vi "output.vi"(8 "error in":errorcluster, 10 "data table in":T1, 11 "SQLite runtime in":refnum<class "SQLite runtime.lvclass">) -> (0 "error out":errorcluster, 2 "data table out":T1, 3 "SQLite runtime out":refnum<class "SQLite runtime.lvclass">)   [LabVIEW 2014, in "SQLite runtime.lvclass"]
doc: "Provides an interface for writing data to a module at runtime. While this interface performs no operations, a child should provide an override which may write to any open sessions, references, or interfaces."
uses:
  SQLite runtime.lvclass
  <vilib>/NI/Tag Bus/table/data table.ctl
  SQLite runtime.lvclass/SQLite runtime.ctl
  <vilib>/drjdpowell/SQLite Library/SQL Statement/SQL Statement.lvclass/SQL Statement.ctl
  <vilib>/NI/Tag Bus/table/data polymorphs/read one/read Double.vi
  <vilib>/NI/Tag Bus/table/data polymorphs/read one/read Single.vi
  <vilib>/drjdpowell/SQLite Library/SQL Statement/Bind Real.vi
  <vilib>/NI/Tag Bus/table/data polymorphs/read one/read I64.vi
  <vilib>/NI/Tag Bus/table/data polymorphs/read one/read I32.vi
  <vilib>/NI/Tag Bus/table/data polymorphs/read one/read I16.vi
  <vilib>/NI/Tag Bus/table/data polymorphs/read one/read I8.vi
  <vilib>/NI/Tag Bus/table/data polymorphs/read one/read U64.vi
  <vilib>/NI/Tag Bus/table/data polymorphs/read one/read U32.vi
  <vilib>/NI/Tag Bus/table/data polymorphs/read one/read U16.vi
  <vilib>/NI/Tag Bus/table/data polymorphs/read one/read U8.vi
  <vilib>/NI/Tag Bus/table/data polymorphs/read one/read Boolean.vi
  <vilib>/drjdpowell/SQLite Library/SQL Statement/Bind Integer.vi
  <vilib>/NI/Tag Bus/table/data polymorphs/read one/read String.vi
  <vilib>/drjdpowell/SQLite Library/SQL Statement/Bind Text.vi
  <vilib>/drjdpowell/SQLite Library/SQL Statement/First Step.vi
  <vilib>/drjdpowell/SQLite Library/SQL Statement/Reset (Property).vi
  <vilib>/drjdpowell/SQLite Library/SQL Statement/Step.vi
  <vilib>/drjdpowell/SQLite Library/SQL Statement/Reset.vi
  <vilib>/drjdpowell/SQLite Library/SQL Statement/Error Message.vi
  <vilib>/drjdpowell/SQLite Library/SQL Statement/SQL.vi
  <vilib>/NI/Tag Bus/table/data table.lvlib
  <vilib>/drjdpowell/SQLite Library/SQL Statement/SQL Statement.lvclass
panel:
  out "SQL 2":string
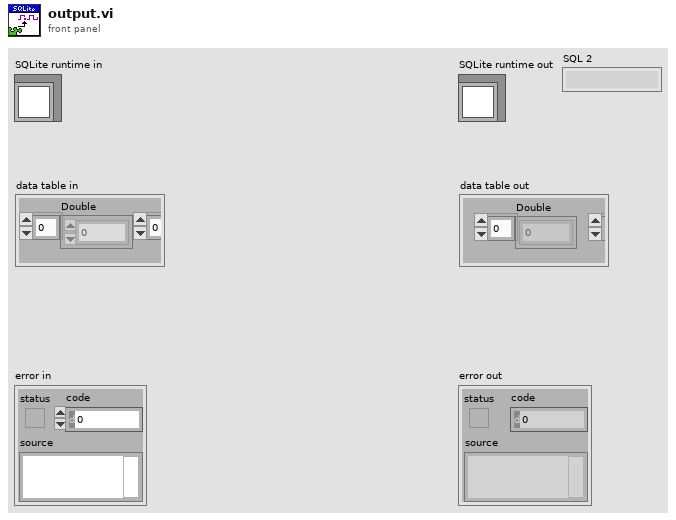
[diagram p1: front panel]
types:
  T1 = typedef "tag bus.lvlib/data table.lvlib/data table.ctl" = cluster{"Double":dbl[], "Single":sgl[], "I64":i64[], "I32":i32[], "I16":i16[], "I8":i8[], "U64":u64[], "U32":u32[], "U16":u16[], "U8":u8[], "Boolean":bool[], "String":string[], "Array of Double":cluster{"DBL Array":dbl[]}[], "Array of Single":cluster{"SGL Array":sgl[]}[], "Array of I64":cluster{"I64 Array":i64[]}[], "Array of I32":cluster{"I32 Array":i32[]}[], "Array of I16":cluster{"I16 Array":i16[]}[], "Array of I8":cluster{"I8 Array":i8[]}[], "Array of U64":cluster{"U64 Array":u64[]}[], "Array of U32":cluster{"U32 Array":u32[]}[], "Array of U16":cluster{"U16 Array":u16[]}[], "Array of U8":cluster{"U8 Array":u8[]}[], "Array of Boolean":cluster{"Boolean Array":bool[]}[], "Array of String":cluster{"String Array":string[]}[]}
  T2 = typedef "SQLite runtime.lvclass/data map.ctl" = cluster{"DCAF Type":T3, "Index":i32, "SQLite Type":T4, "db key":string}
  T3 = typedef "tag bus.lvlib/tag descriptor.lvclass/Data Type.ctl" = enum16{"Double", "Single", "I64", "I32", "I16", "I8", "U64", "U32", "U16", "U8", "Boolean", "String", "Array of Double", "Array of Single", "Array of I64", "Array of I32", "Array of I16", "Array of I8", "Array of U64", "Array of U32", "Array of U16", "Array of U8", "Array of Boolean", "Array of String"}
  T4 = typedef "SQLite runtime.lvclass/sqlite type.ctl" = enum16{"DBL", "I64", "String"}
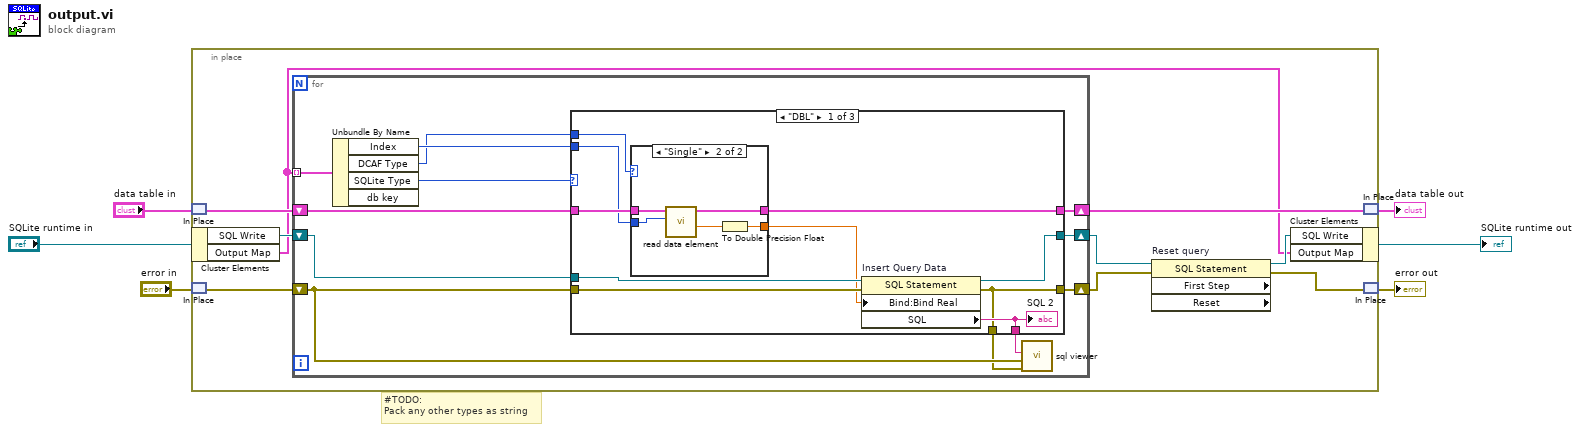
[diagram p0: block diagram]
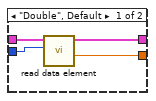
[diagram p2: hidden frame]
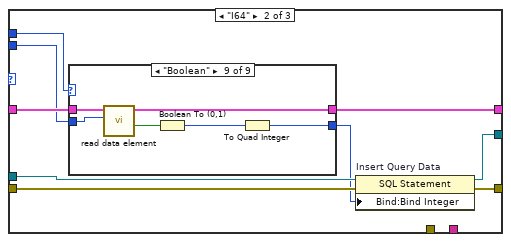
[diagram p3: hidden frame]
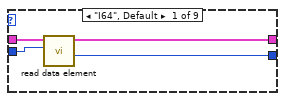
[diagram p4: hidden frame]
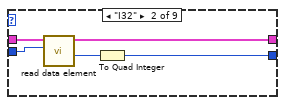
[diagram p5: hidden frame]
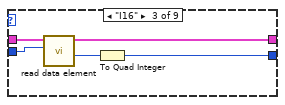
[diagram p6: hidden frame]
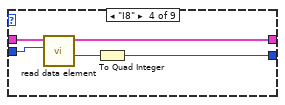
[diagram p7: hidden frame]
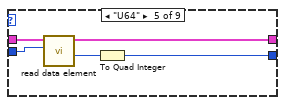
[diagram p8: hidden frame]
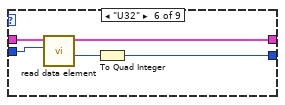
[diagram p9: hidden frame]
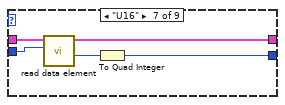
[diagram p10: hidden frame]
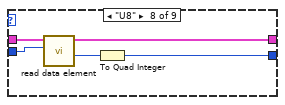
[diagram p11: hidden frame]
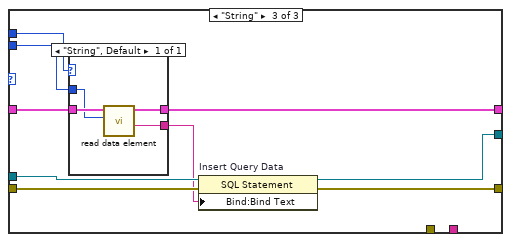
[diagram p12: hidden frame]
diagram:
  # "#TODO:\nPack any other types as string"
  n1 = in-place {
    n2 = in-place-match #1("data table in") -> (w11:T1)
    n3 = in-place-cluster #2("SQLite runtime in") -> ("SQL Write"=w15:refnum<class "SQL Statement.lvclass">, "Output Map"=w9:T2[])
    n4 = in-place-match #3("error in") -> (w14:errorcluster)
    n5 = for {
      shift-right: [w20] -> w7
      shift-left: w15 -> [w19]
      shift-right: [w21] -> w8
      shift-left: w14 -> [w18]
      shift-right: [w23] -> w10
      shift-left: w11 -> [w24]
      tunnel: w9 -> [w27] mode=indexing
      n6 = Unbundle By Name(w27) -> ("Index"=w25:i32, "DCAF Type"=w22:T3, "SQLite Type"=w26:T4)  [unwired: 1 out]
      n7 = case shown="\"DBL\"" w26 {
        tunnel: w19 -> [w37 w55 w109]
        tunnel: [w36 w48 w108] -> w20
        tunnel: w18 -> [w35 w54 w107]
        tunnel: [w28 w53 w106] -> w21
        tunnel: w25 -> [w31 w49 w103]
        tunnel: w24 -> [w34 w52 w105]
        tunnel: [w33 w51 w104] -> w23
        tunnel: w22 -> [w32 w50 w102]
        tunnel: [w29 _ _] -> w17
        tunnel: [w28 _ _] -> w16
        frame "DBL" {
          n8 = case shown="\"Single\"" w32 {
            tunnel: w34 -> [w41 w46]
            tunnel: [w40 w45] -> w33
            tunnel: w31 -> [w39 w44]
            tunnel: [w38 w42] -> w30
            frame "Double", Default {
              n9 = call-poly <vilib>:"read data element.vi"("index"=w39, "data table in"=w41) -> ("value"=w38:dbl, "data table out"=w40:T1)  [unwired: 8 in]
            }
            frame "Single" {
              n10 = call-poly <vilib>:"read data element.vi"("index"=w44, "data table in"=w46) -> ("value"=w43:sgl, "data table out"=w45:T1)  [unwired: 8 in]
              n11 = To Double Precision Float(number=w43) -> (double precision float=w42:dbl)
            }
          }
          n12 = property on="Insert Query Data" class="SQL Statement"(reference=w37, error in=w35, "Bind:Bind Real"=w30) -> (reference out=w36:refnum<class "SQL Statement.lvclass">, error out=w28:errorcluster, "SQL"=w29:string)
          "SQL 2" <- w29
        }
        frame "I64" {
          n13 = case shown="\"Boolean\"" w50 {
            tunnel: w52 -> [w59 w64 w69 w74 w79 w84 w89 w94 w100]
            tunnel: [w58 w63 w68 w73 w78 w83 w88 w93 w99] -> w51
            tunnel: w49 -> [w57 w62 w67 w72 w77 w82 w87 w92 w98]
            tunnel: [w56 w60 w65 w70 w75 w80 w85 w90 w95] -> w47
            frame "I64", Default {
              n14 = call-poly <vilib>:"read data element.vi"("index"=w57, "data table in"=w59) -> ("value"=w56:i64, "data table out"=w58:T1)  [unwired: 8 in]
            }
            frame "I32" {
              n15 = call-poly <vilib>:"read data element.vi"("index"=w62, "data table in"=w64) -> ("value"=w61:i32, "data table out"=w63:T1)  [unwired: 8 in]
              n16 = To Quad Integer(1:w61) -> (0:w60:i64)
            }
            frame "I16" {
              n17 = call-poly <vilib>:"read data element.vi"("index"=w67, "data table in"=w69) -> ("value"=w66:i16, "data table out"=w68:T1)  [unwired: 8 in]
              n18 = To Quad Integer(1:w66) -> (0:w65:i64)
            }
            frame "I8" {
              n19 = call-poly <vilib>:"read data element.vi"("index"=w72, "data table in"=w74) -> ("value"=w71:i8, "data table out"=w73:T1)  [unwired: 8 in]
              n20 = To Quad Integer(1:w71) -> (0:w70:i64)
            }
            frame "U64" {
              n21 = call-poly <vilib>:"read data element.vi"("index"=w77, "data table in"=w79) -> ("value"=w76:u64, "data table out"=w78:T1)  [unwired: 8 in]
              n22 = To Quad Integer(1:w76) -> (0:w75:i64)
            }
            frame "U32" {
              n23 = call-poly <vilib>:"read data element.vi"("index"=w82, "data table in"=w84) -> ("value"=w81:u32, "data table out"=w83:T1)  [unwired: 8 in]
              n24 = To Quad Integer(1:w81) -> (0:w80:i64)
            }
            frame "U16" {
              n25 = call-poly <vilib>:"read data element.vi"("index"=w87, "data table in"=w89) -> ("value"=w86:u16, "data table out"=w88:T1)  [unwired: 8 in]
              n26 = To Quad Integer(1:w86) -> (0:w85:i64)
            }
            frame "U8" {
              n27 = call-poly <vilib>:"read data element.vi"("index"=w92, "data table in"=w94) -> ("value"=w91:u8, "data table out"=w93:T1)  [unwired: 8 in]
              n28 = To Quad Integer(1:w91) -> (0:w90:i64)
            }
            frame "Boolean" {
              n29 = call-poly <vilib>:"read data element.vi"("index"=w98, "data table in"=w100) -> ("value"=w97:bool, "data table out"=w99:T1)  [unwired: 8 in]
              n30 = Boolean To (0,1)(Boolean=w97) -> (0, 1=w96:i16)
              n31 = To Quad Integer(1:w96) -> (0:w95:i64)
            }
          }
          n32 = property on="Insert Query Data" class="SQL Statement"(reference=w55, error in=w54, "Bind:Bind Integer"=w47) -> (reference out=w48:refnum<class "SQL Statement.lvclass">, error out=w53:errorcluster)
        }
        frame "String" {
          n33 = case shown="\"String\", Default" w102 {
            tunnel: w105 -> [w113]
            tunnel: [w112] -> w104
            tunnel: w103 -> [w111]
            tunnel: [w110] -> w101
            frame "String", Default {
              n34 = call-poly <vilib>:"read data element.vi"("index"=w111, "data table in"=w113) -> ("value"=w110:string, "data table out"=w112:T1)  [unwired: 8 in]
            }
          }
          n35 = property on="Insert Query Data" class="SQL Statement"(reference=w109, error in=w107, "Bind:Bind Text"=w101) -> (reference out=w108:refnum<class "SQL Statement.lvclass">, error out=w106:errorcluster)
        }
      }
      n36 = call "sql viewer.vi"("error in (no error) 2"=w16, "error in (no error)"=w18, "SQL2"=w17) -> ()  [unwired: 9 in]
    }
    n37 = property on="Reset query" class="SQL Statement" props=["First Step", "Reset"](reference=w7, error in=w8) -> (reference out=w13:refnum<class "SQL Statement.lvclass">, error out=w12:errorcluster)  [unwired: 2 out]
    n38 = in-place-cluster #2("SQL Write"=w13, "Output Map"=w9) -> (→"SQLite runtime out":refnum<class "SQLite runtime.lvclass">)
    n39 = in-place-match #1(w10) -> (→"data table out":T1)
    n40 = in-place-match #3(w12) -> (→"error out":errorcluster)
  }
